vi "Get or Init RHS Class.vi"(5 "type check? (T)":bool=TRUE, 7 "target RHS":refnum<class "NI_RHS.lvclass">, 8 "error in (no error)":errorcluster, 11 "PDE out":refnum<class "NI_PDE.lvclass">) -> (0 "error out":errorcluster, 2 "RHS out":refnum<class "NI_RHS.lvclass">, 3 "PDE in":refnum<class "NI_PDE.lvclass">)   [LabVIEW 2020, in "NI_PDE.lvlib" / "NI_PDE.lvclass"]
uses:
  <vilib>/gmath/pde.llb/PDEClass/NI_PDE.lvclass
  <vilib>/gmath/pde.llb/RHSClass/NI_RHS.lvclass
  <vilib>/gmath/pde.llb/RHSClass/Class Type.ctl
  <vilib>/gmath/pde.llb/Common/PDE_Error.ctl
  <vilib>/gmath/NI_PDE.lvlib
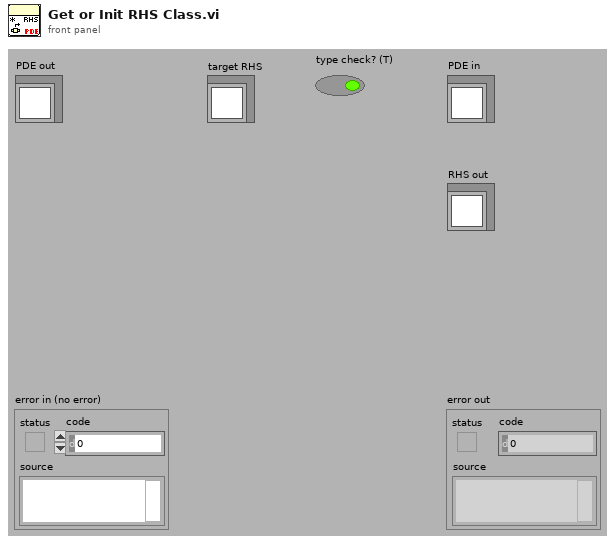
[diagram p1: front panel]
types:
  T1 = typedef "NI_PDE.lvlib/PDE_Error.ctl" = enum16{"No Error", "k is zero", "End point <= start point", "# of time steps < 2", "# of spatial points < 3", "# of grid < 1 for FEM", "# of boundary < 3 for FEM", "Incompatible RHS size", "Incompatible BC size", "Incompatible IC size", "PDE class conflict", "RHS class conflict", "Domain class conflict", "BC class conflict", "IC class conflict"}
  T2 = typedef "NI_PDE.lvlib/NI_RHS.lvclass/Class Type.ctl" = i32
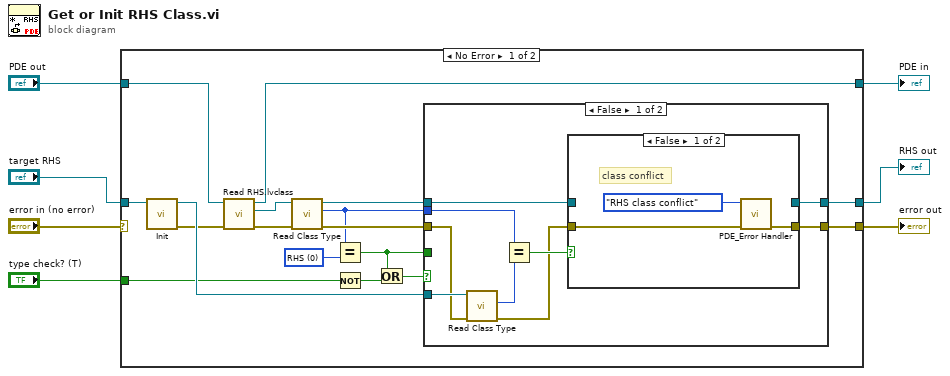
[diagram p0: block diagram]
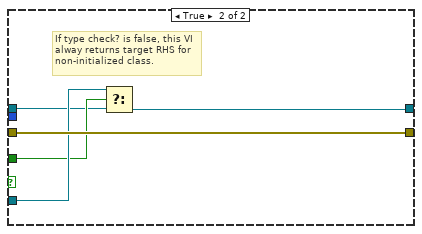
[diagram p3: hidden frame]
diagram:
  n1 = case shown="No Error" "error in (no error)" {
    selector: "error in (no error)" -> [_ w46]
    tunnel: "PDE out" -> [w24 w44]
    tunnel: [w17 w45] -> w6
    tunnel: [w16 w46] -> w5
    tunnel: [w15 w44] -> w4
    tunnel: "target RHS" -> [w14 w45]
    tunnel: "type check? (T)" -> [w10 _]
    frame No Error {
      w21 = T2 0 items=["RHS"=0, "RHS_2D"=20, "RHS_2D_Numeric"=21, "RHS_2D_VIRef"=22, "RHS_3D"=30, "RHS_3D_Numeric"=31, "RHS_3D_VIRef"=32] ("y")
      n2 = call-dynamic "Init.vi"("RHS"=w14) -> ("error out"=w12:errorcluster, "initialized RHS"=w13:refnum<class "NI_RHS.lvclass">)  [unwired: 1 in, 8 out]
      n3 = call-dynamic "Read RHS.lvclass.vi"("error in (no error)"=w12, "PDE.lvclass in"=w24) -> ("error out"=w22:errorcluster, "RHS.lvclass"=w23:refnum<class "NI_RHS.lvclass">, "PDE.lvclass out"=w15:refnum<class "NI_PDE.lvclass">)  [unwired: 7 out]
      n4 = call-dynamic "Read Class Type.vi"("error in (no error)"=w22, "RHS.lvclass in"=w23) -> ("error out"=w19:errorcluster, "RHS class type"=w18:T2, "RHS.lvclass out"=w20:refnum<class "NI_RHS.lvclass">)  [unwired: 7 out]
      n5 = Equal?(x=w18, y=w21) -> (x = y?=w8:bool)
      n6 = Not(x=w10) -> (.not. x?=w9:bool)
      n7 = Or(x=w8, y=w9) -> (x .or. y?=w11:bool)
      n8 = case shown="False" w11 {
        tunnel: w20 -> [w32 w40]
        tunnel: w19 -> [w26 w43]
        tunnel: [w30 w39] -> w17
        tunnel: w18 -> [w31 _]
        tunnel: [w29 w43] -> w16
        tunnel: w13 -> [w28 w42]
        tunnel: w8 -> [_ w41]
        frame False {
          n9 = call-dynamic "Read Class Type.vi"("error in (no error)"=w26, "RHS.lvclass in"=w28) -> ("error out"=w25:errorcluster, "RHS class type"=w27:T2)  [unwired: 8 out]
          n10 = Equal?(x=w31, y=w27) -> (x = y?=w33:bool)
          n11 = case shown="False" w33 {
            tunnel: w25 -> [w35 w37]
            tunnel: w32 -> [_ w38]
            tunnel: [_ w38] -> w30
            tunnel: [w34 w37] -> w29
            frame False {
              # "class conflict"
              n12 = call <vilib>:"PDE_Error Handler.vi"("error in (no error)"=w35, "PDE error"=PDE_Error."RHS class conflict") -> ("error out"=w34:errorcluster)  [unwired: 9 out]
            }
            frame True {
            }
          }
        }
        frame True {
          # "If type check? is false, this VI alway returns target RHS for non-initialized class."
          n13 = Select(t=w42, s=w41, f=w40) -> (s? t:f=w39:refnum<class "NI_RHS.lvclass">)
        }
      }
    }
    frame Error {
    }
  }
  "RHS out" <- w6
  "error out" <- w5
  "PDE in" <- w4
